vi "JoystickPlayer.vi"(6 "error in":errorcluster) -> ()   [LabVIEW 2014]
uses:
  <vilib>/Analysis/Matrix/Datatypes/RealMatrix.ctl
  Automated Tasks/AutomationGlobals.vi
  <vilib>/Analysis/Matrix/NI_Matrix.lvlib
panel:
  in  "JoystickRecorded":T1=array4x2273[9092 elements]
  in  "GantryButtonsOut":T1
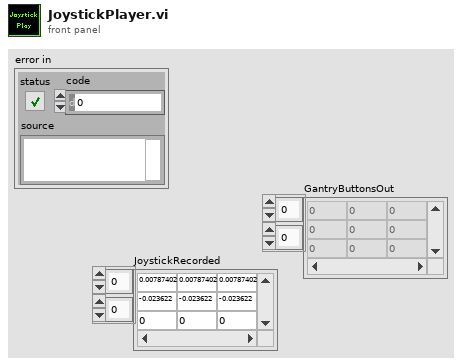
[diagram p1: front panel]
types:
  T1 = typedef "NI_Matrix.lvlib/RealMatrix.ctl" = dbl[][]
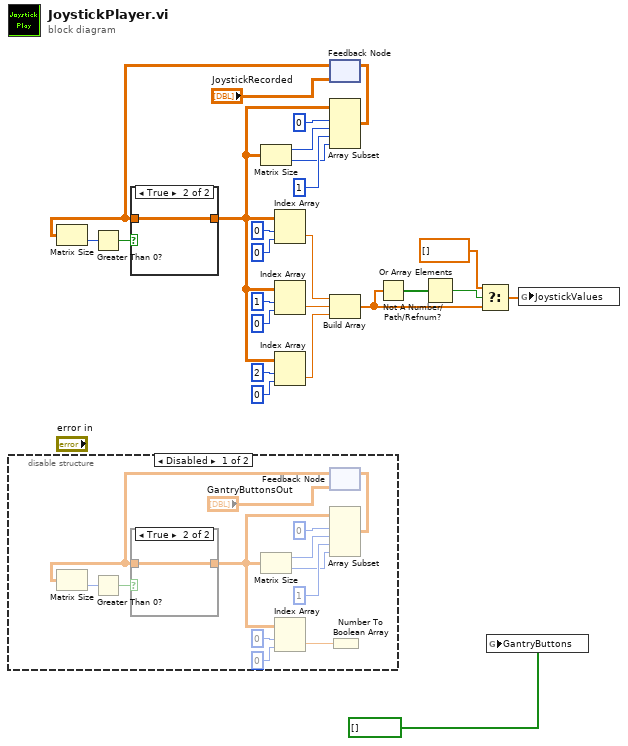
[diagram p0: block diagram]
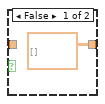
[diagram p2: hidden frame]
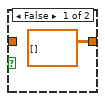
[diagram p4: hidden frame]
diagram:
  n1 = disable-structure shown="Disabled" {
    frame Disabled {
      n2 = feedback #1("GantryButtonsOut") -> (w28:T1)
      n3 = Matrix Size(0:w28) -> (2:w31:i32)  [unwired: 1 out]
      n4 = Greater Than 0?(x=w31) -> (x > 0?=w30:bool)
      n5 = case shown="True" w30 {
        tunnel: w28 -> [_ w40]
        tunnel: [T1 [] ("JoystickRecorded") w40] -> w29
        frame False {
        }
        frame True {
        }
      }
      n6 = Matrix Size(0:w29) -> (1:w36:i32, 2:w35:i32)
      n7 = Index Array(array=w29, index (row)=0, index (col)=0) -> (element=w27:dbl)
      n8 = Array Subset(array=w29, index (row)=0 ("row 1"), length (row)=w36, index (col)=1 ("column 1"), length (col)=w35) -> (w32:T1)
      n9 = feedback-in #1(w32) -> ()
      n10 = Number To Boolean Array(number=w27) -> ()  [unwired: 1 out]
    }
    frame Enabled {
    }
  }
  n11 = feedback #2("JoystickRecorded") -> (w9:T1)
  n12 = Matrix Size(0:w9) -> (2:w11:i32)  [unwired: 1 out]
  n13 = Greater Than 0?(x=w11) -> (x > 0?=w10:bool)
  n14 = case shown="True" w10 {
    tunnel: w9 -> [_ w42]
    tunnel: [T1 [] ("JoystickRecorded") w42] -> w8
    frame False {
    }
    frame True {
    }
  }
  n15 = Matrix Size(0:w8) -> (1:w23:i32, 2:w22:i32)
  n16 = Index Array(array=w8, index (row)=0, index (col)=0) -> (element=w19:dbl)
  n17 = Index Array(array=w8, index (row)=1, index (col)=0) -> (element=w14:dbl)
  n18 = Index Array(array=w8, index (row)=2, index (col)=0) -> (element=w13:dbl)
  n19 = Array Subset(array=w8, index (row)=0 ("row 1"), length (row)=w23, index (col)=1 ("column 1"), length (col)=w22) -> (w12:T1)
  n20 = feedback-in #2(w12) -> ()
  n21 = Build Array(w19, w14, w13) -> (w3:dbl[])
  n22 = Not A Number/Path/Refnum?(number/path/refnum=w3) -> (NaN/Path/Refnum?=w6:bool[])
  n23 = Or Array Elements(Boolean array=w6) -> (logical OR=w5:bool)
  n24 = Select(t=dbl[] [] ("f"), s=w5, f=w3) -> (s? t:f=w7:dbl[])
  n25 = global write "AutomationGlobals.vi" "GantryButtons"(bool[] [] ("Boolean array")) -> ()
  n26 = global write "AutomationGlobals.vi" "JoystickValues"(w7) -> ()
